vi "Read Spec Page Path.vi"(8 "error in (no error)":errorcluster, 11 "myRIOMetaDataObj in":refnum<class "myRIOMetaDataObj.lvclass">) -> (0 "error out":errorcluster, 2 "Path to Spec Page VI":path, 3 "myRIOMetaDataObj out":refnum<class "myRIOMetaDataObj.lvclass">)   [LabVIEW 2021, in "myRIOMetaDataObj.lvclass"]
uses:
  myRIOMetaDataObj.lvclass
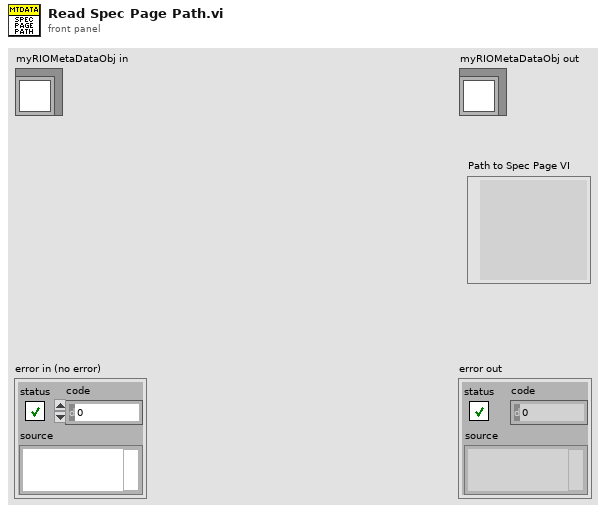
[diagram p1: front panel]
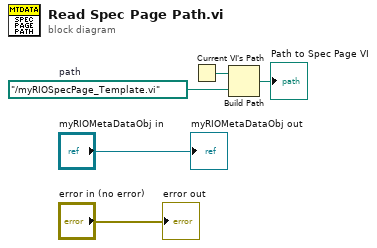
[diagram p0: block diagram]
diagram:
  w4 = path "../myRIOSpecPage_Template.vi"  # path
  n1 = Current VI's Path() -> (path=w5:path)
  n2 = Build Path(base path=w5, name or relative path=w4) -> (appended path=→"Path to Spec Page VI":path)
  "error out" <- "error in (no error)"
  "myRIOMetaDataObj out" <- "myRIOMetaDataObj in"
